vi "CRYCheck Main Generator.vi"(11 "Gen Idx":i32) -> (3 "Is Main?":bool)   [LabVIEW 2013]
uses:
  CRYMisc vis settings global.vi
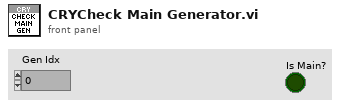
[diagram p1: front panel]
types:
  T1 = cluster{"Gen Idx":i32, "Chn Idx":i32, "Data":sgl[]}[]
  T2 = cluster{"Gen Idx":i32, "Chn Idx":i32, "Data":sgl[]}
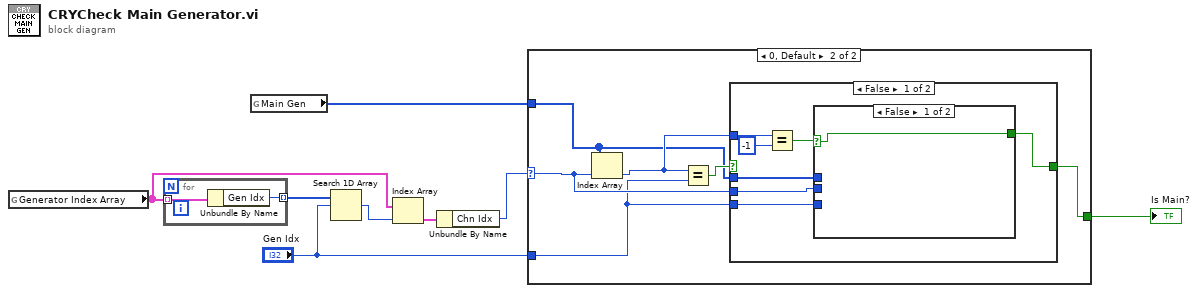
[diagram p0: block diagram]
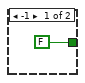
[diagram p2: hidden frame]
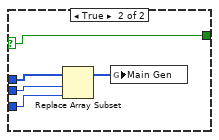
[diagram p3: hidden frame]
diagram:
  n1 = global read "CRYMisc vis settings global.vi" "Generator Index Array"() -> (w3:T1)
  n2 = for {
    tunnel: w3 -> [w10] mode=indexing
    tunnel: [w9] -> w6 mode=indexing
    n3 = Unbundle By Name(w10) -> ("Gen Idx"=w9:i32)
  }
  n4 = global read "CRYMisc vis settings global.vi" "Main Gen"() -> (w7:i32[])
  n5 = Search 1D Array(1D array=w6, element="Gen Idx") -> (index of element=w4:i32)  [unwired: 1 in]
  n6 = Index Array(array=w3, index=w4) -> (element=w2:T2)
  n7 = Unbundle By Name(w2) -> ("Chn Idx"=w1:i32)
  n8 = case shown="0, Default" w1 {
    selector: w1 -> [_ w13]
    tunnel: [FALSE w16] -> w8
    tunnel: w7 -> [_ w14]
    tunnel: "Gen Idx" -> [_ w12]
    frame -1 {
    }
    frame 0, Default {
      n9 = Index Array(array=w14, index=w13) -> (element=w15:i32)
      n10 = Equal?(x=w15, y=w12) -> (x = y?=w17:bool)
      n11 = case shown="False" w17 {
        selector: w17 -> [_ w31]
        tunnel: [w21 w31] -> w16
        tunnel: w15 -> [w24 _]
        tunnel: w14 -> [w20 _]
        tunnel: w13 -> [w19 _]
        tunnel: w12 -> [w18 _]
        frame False {
          n12 = Equal?(x=w24, y=-1) -> (x = y?=w22:bool)
          n13 = case shown="False" w22 {
            selector: w22 -> [w25 w30]
            tunnel: [w25 w30] -> w21
            tunnel: w20 -> [_ w29]
            tunnel: w19 -> [_ w28]
            tunnel: w18 -> [_ w27]
            frame False {
            }
            frame True {
              n14 = Replace Array Subset(array=w29, new element=w27, index=w28) -> (w26:i32[])
              n15 = global write "CRYMisc vis settings global.vi" "Main Gen"(w26) -> ()
            }
          }
        }
        frame True {
        }
      }
    }
  }
  "Is Main?" <- w8
